vi "Dialog_FileInUse.vi"(11 "Path":path) -> (3 "Cancelled":bool)   [LabVIEW 2012]
panel:
  out "Path 2":path
  in  "Cancel Button":bool
  in  "Try Again":bool
  # "File in use!"
  # "Close the file and try again"
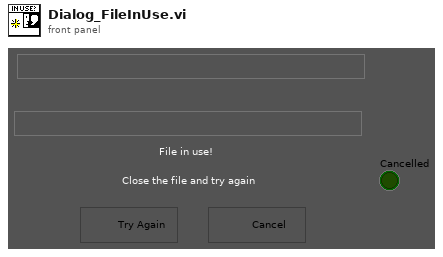
[diagram p1: front panel]
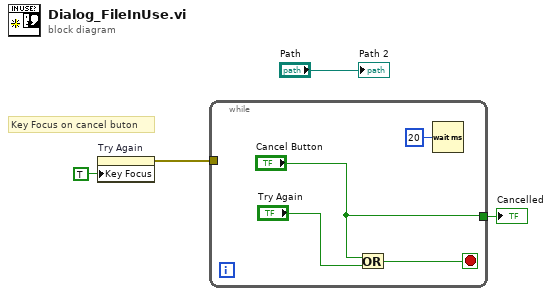
[diagram p0: block diagram]
diagram:
  # "Key Focus on cancel buton"
  n1 = property on="Try Again" class="Bool"("Key Focus"=TRUE) -> (error out=w1:errorcluster)  [unwired: 2 in, 1 out]
  n2 = while {
    tunnel: ["Cancel Button"] -> w4
    tunnel: w1 -> [_]
    stop <- w7 stop-if-true
    n3 = Or(x="Cancel Button", y="Try Again") -> (x .or. y?=w7:bool)
    n4 = Wait (ms)(milliseconds to wait=u32 20) -> ()  [unwired: 1 out]
  }
  "Cancelled" <- w4
  "Path 2" <- "Path"
